vi "systemExec_bat.vi"() -> ()   [LabVIEW 2012]
panel:
  out "return code":i32
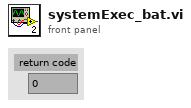
[diagram p1: front panel]
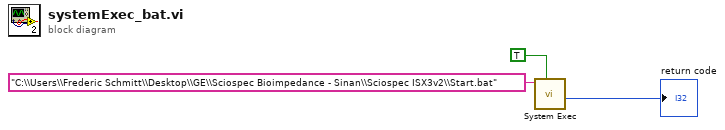
[diagram p0: block diagram]
diagram:
  n1 = call <vilib>:"System Exec.vi"("wait until completion? (T)"=TRUE, "command line"="C:\\Users\\Frederic Schmitt\\Desktop\\GE\\Sciospec Bioimpedance - Sinan\\Sciospec ISX3v2\\Start.bat") -> ("return code"=→"return code":i32)  [unwired: 6 in, 3 out]
